vi "Process.vi"(8 "error in":errorcluster, 11 "UI_Main_Test":refnum<class "UI_Main.lvclass">) -> (0 "error out":errorcluster, 3 "UI_Main_Test out":refnum<class "UI_Main.lvclass">)   [LabVIEW 2016, in "UI_Main.lvclass"]
doc: "---------------------------------------------------------------\nJKI State Machine Objects™\nhttp://jki.net/state-machine-objects/\nCopyright (C) 2005-2015, JKI <info@jki.net>\nALL RIGHTS RESERVED"
uses:
  UI_Main.lvclass
  <vilib>/JKI/JKI SMO/SMO/SMO.lvclass
  <vilib>/JKI/JKI SMO/SMO/Typedefs/Parent Call--Enum.ctl
  UI_DAQ_config/UI_DAQ_config.lvclass
  Typedefs/SubUIs.ctl
  UI_Scope/UI_Scope.lvclass
  UI_Generator_Config/UI_Generator_Config.lvclass
  UI_DSP_Config/UI_DSP_Config.lvclass
  lockin/system.lvclass
  C:/Program Files (x86)/National Instruments/LabVIEW 2016/vi.lib/JKI/JKI SMO/SMO/SMO.lvclass
panel:
  in  "config Generator":bool
  in  "Shutdown":bool
  in  "config DSP":bool
  in  "config DAQs":bool
  in  "show Scope":bool
  # "For instructions on how to use the JKI State Machine Objects, examples and video tutorials, visit:\nhttp://jki.net/state-machine-objects/\n\nJKI State Machine Objects™\nhttp://jki.net/state-machine-objects/\nCopyright (C) 2005-2015, JKI <info@jki.net>\nALL RIGHTS RESERVED"
  # "main UI: Always running?"
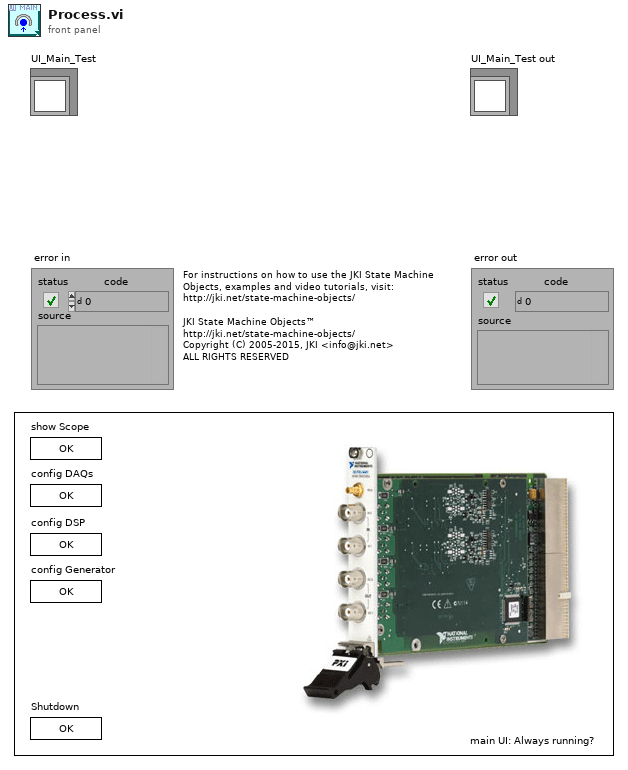
[diagram p1: front panel]
types:
  T1 = typedef "SMO.lvclass/Parent Call--Enum.ctl" = enum16{"Allows parent to run", "Does not request parent to run"}
  T2 = enum32{"invalid app kind", "Development System", "Run Time System", "Student Edition", "Embedded LabVIEW", "Evaluation", "Custom"}
  T3 = enum32{"Invalid", "Standard", "Closed", "Hidden", "Minimized", "Maximized"}
  T4 = enum32{"Bad", "Idle", "Run top level", "Running"}
  T5 = typedef "system.lvclass/Dependencies-cluster.ctl" = cluster{"DAQ_Manager":refnum<class "DAQ_Manager.lvclass">, "DSP":refnum<class "DSP.lvclass">, "Generator":refnum<class "Generator.lvclass">, "Scope":refnum<class "Scope.lvclass">}
  T6 = typedef "UI_Main.lvclass/SubUIs.ctl" = cluster{"UI_DAQ":refnum<class "UI_DAQ_config.lvclass">, "UI_DSP":refnum<class "UI_DSP_Config.lvclass">, "UI_Generator":refnum<class "UI_Generator_Config.lvclass">, "UI_Scope":refnum<class "UI_Scope.lvclass">}
  T7 = cluster{"Core":cluster{"Current VI Reference":refnum<vi>, "Close Panel on Exit?":bool, "error":errorcluster}, "Self Reference":refnum<class "UI_Main.lvclass">, "system":refnum<class "system.lvclass">, "Dependencies":T5, "UIs":T6}
  T8 = cluster{"Current VI Reference":refnum<vi>, "Close Panel on Exit?":bool, "error":errorcluster}
  T9 = typedef "SMO.lvclass/Protected Events.ctl" = cluster{"StopProcesses":refnum<user-event>, "AbortProcesses":refnum<user-event>, "Config Changed":refnum<user-event>, "Dependency":refnum<user-event>}
  T10 = typedef "SMO.lvclass/SMOState --Enum.ctl" = enum16{"unknown", "Created", "Started", "Stopped"}
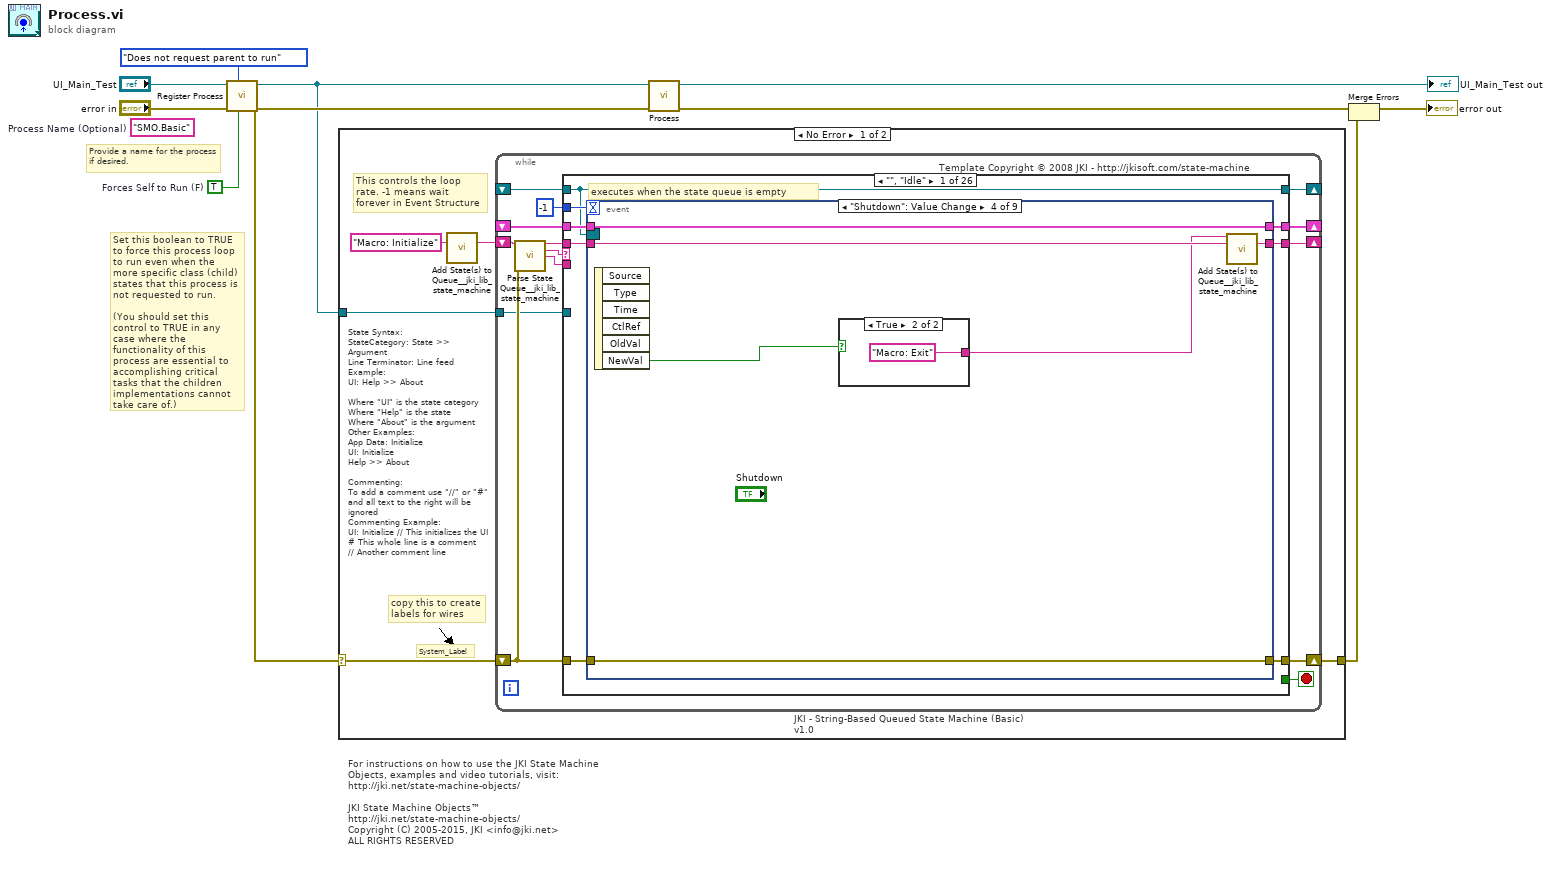
[diagram p0: block diagram]
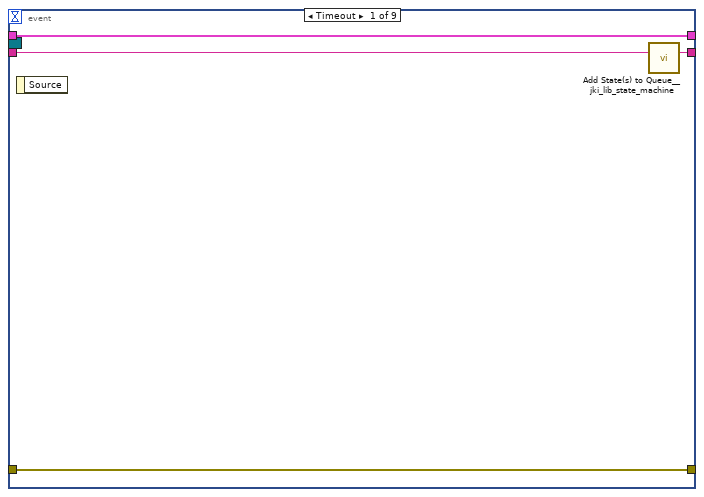
[diagram p2: hidden frame]
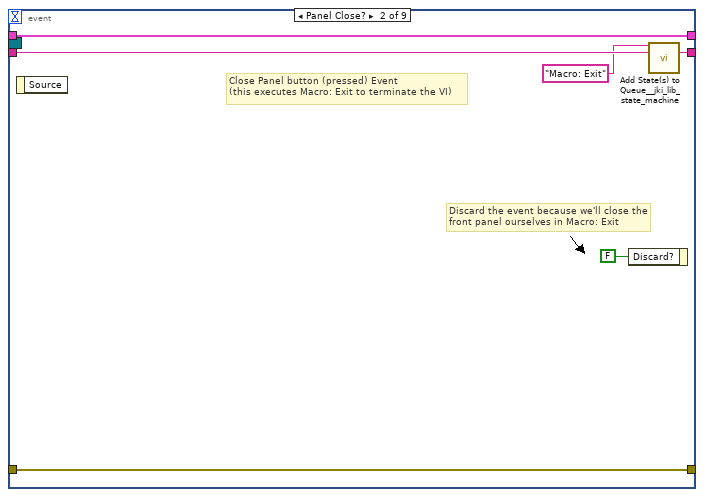
[diagram p3: hidden frame]
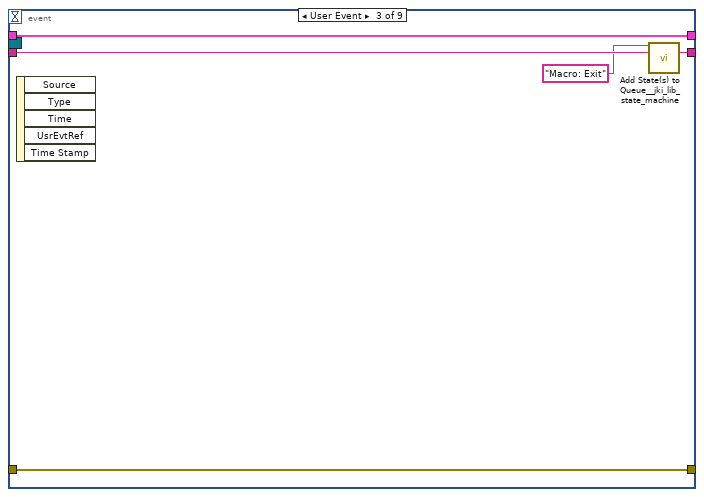
[diagram p4: hidden frame]
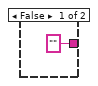
[diagram p5: hidden frame]
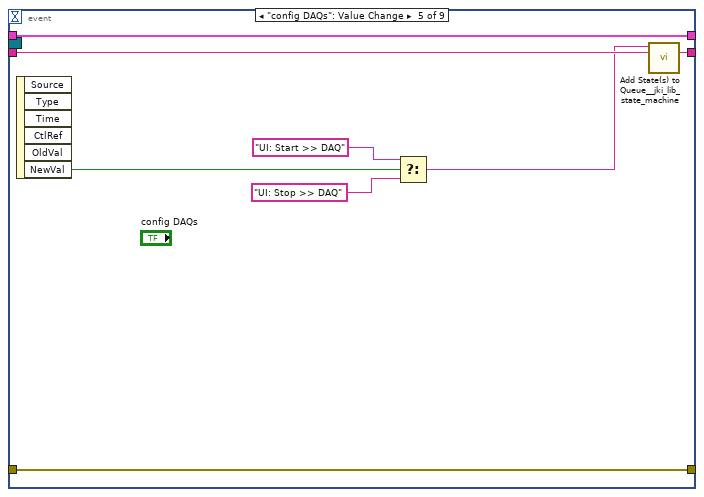
[diagram p6: hidden frame]
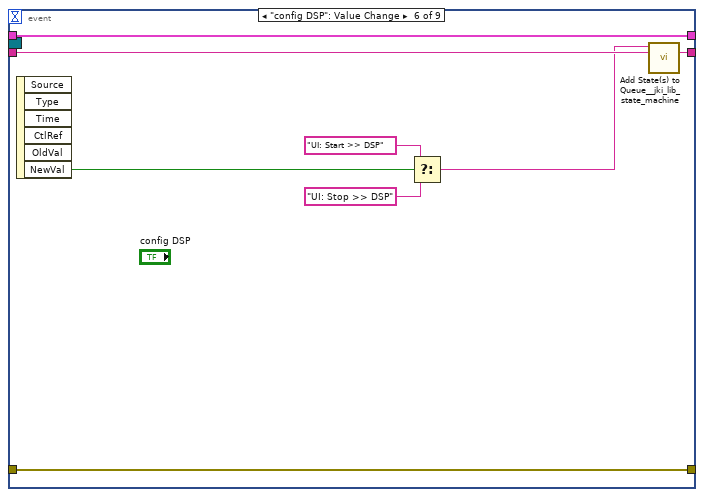
[diagram p7: hidden frame]
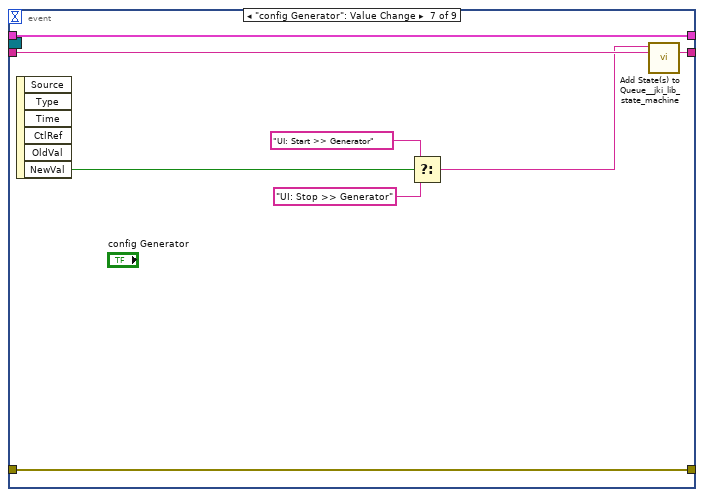
[diagram p8: hidden frame]
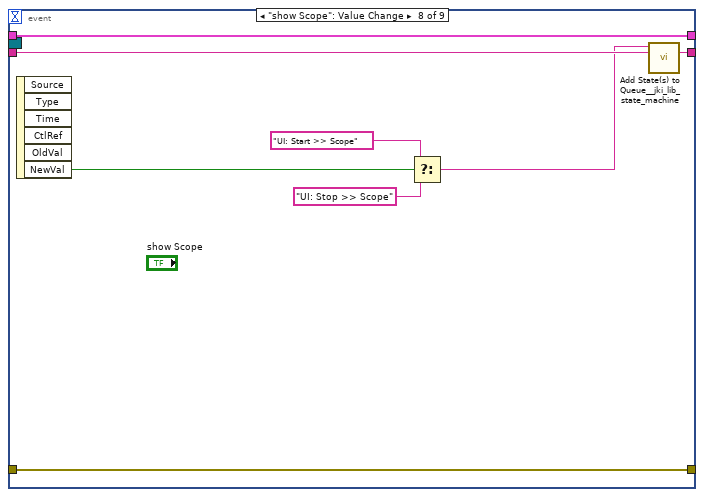
[diagram p9: hidden frame]
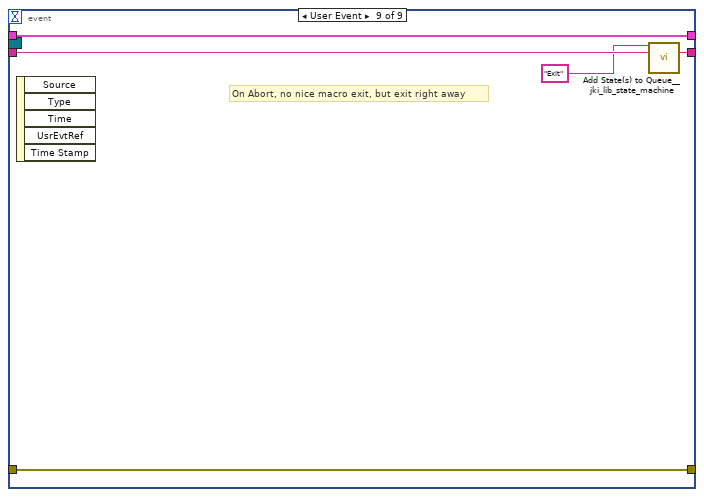
[diagram p10: hidden frame]
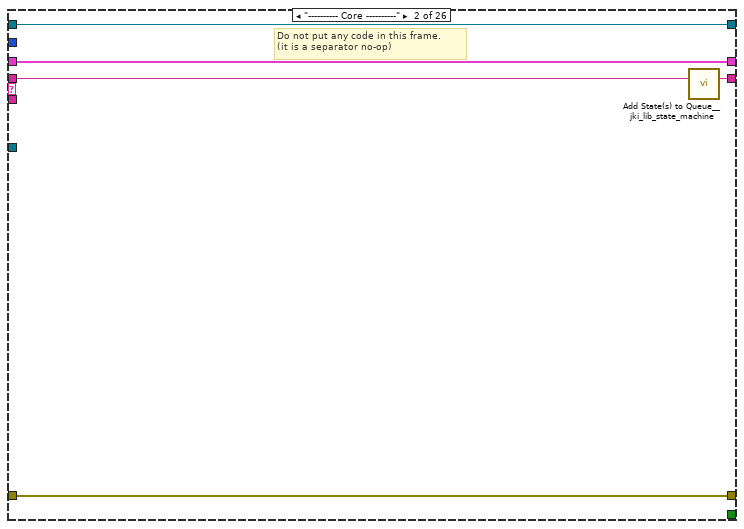
[diagram p11: hidden frame]
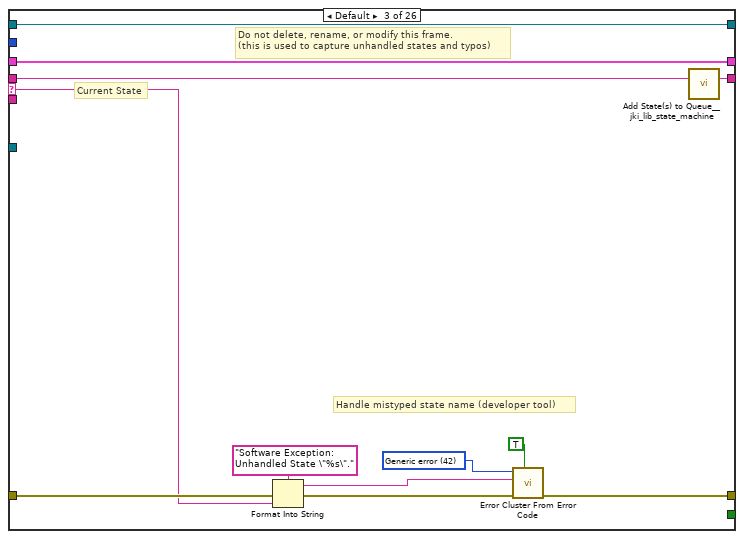
[diagram p12: hidden frame]
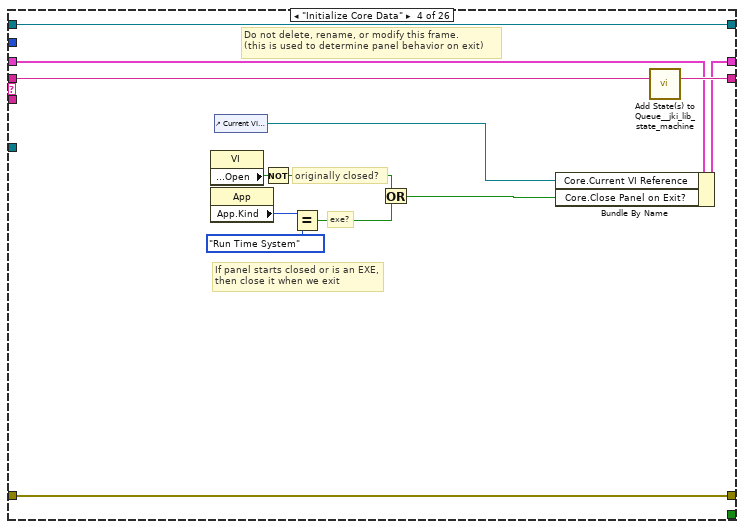
[diagram p13: hidden frame]
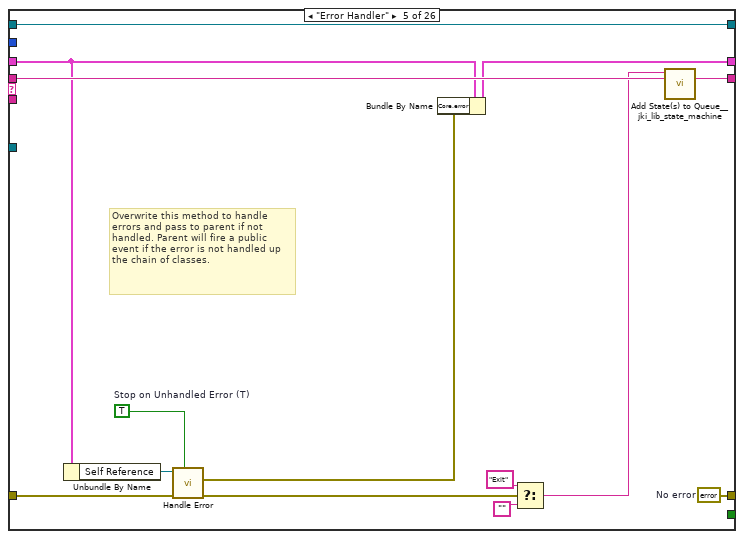
[diagram p14: hidden frame]
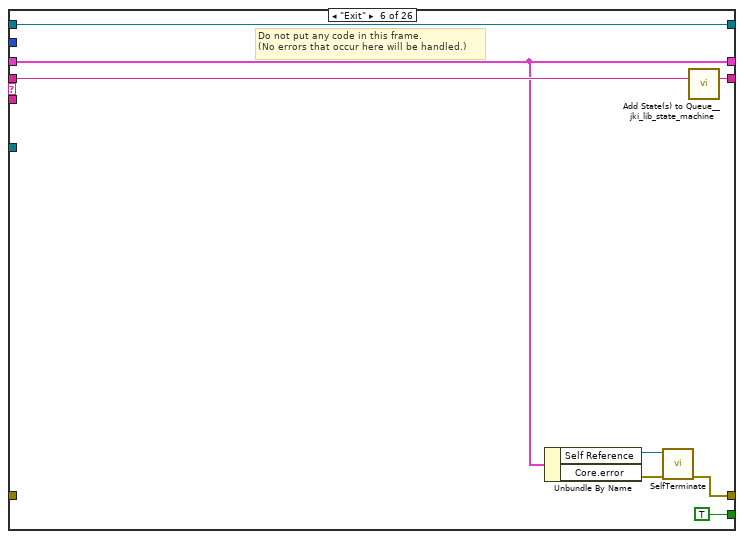
[diagram p15: hidden frame]
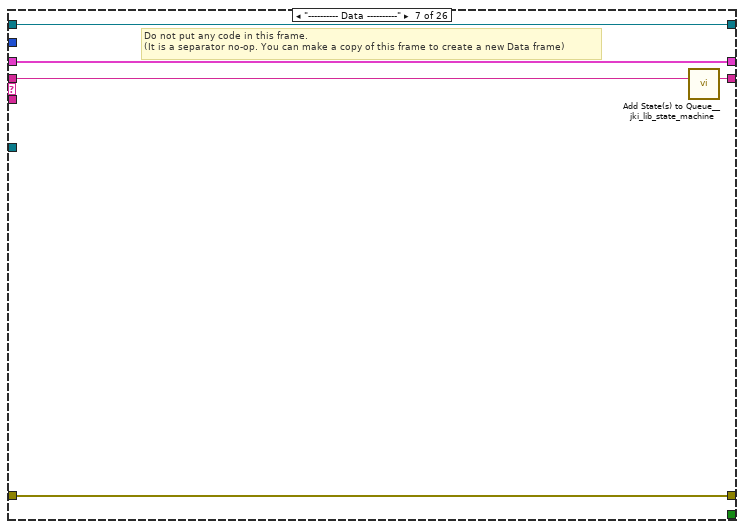
[diagram p16: hidden frame]
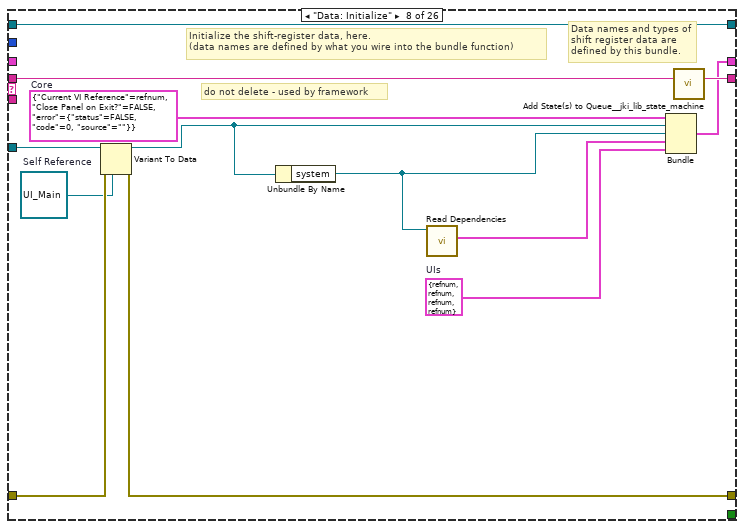
[diagram p17: hidden frame]
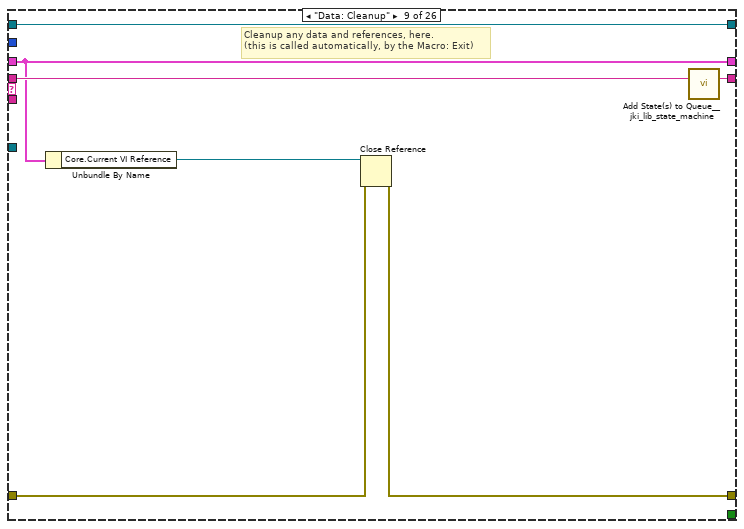
[diagram p18: hidden frame]
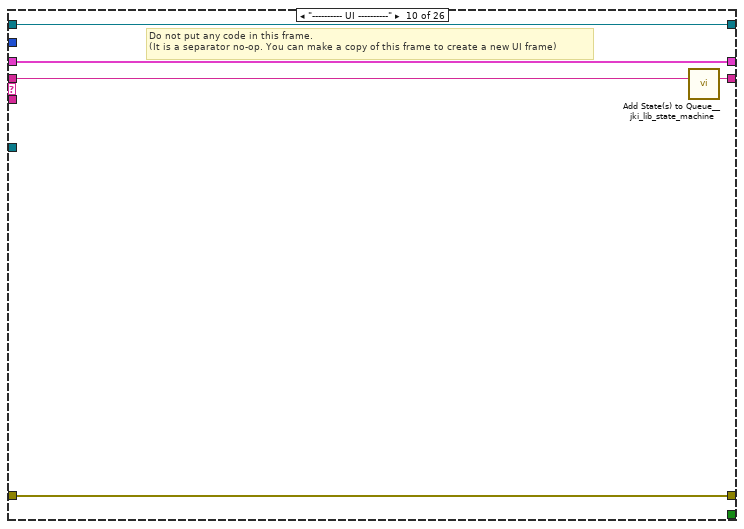
[diagram p19: hidden frame]
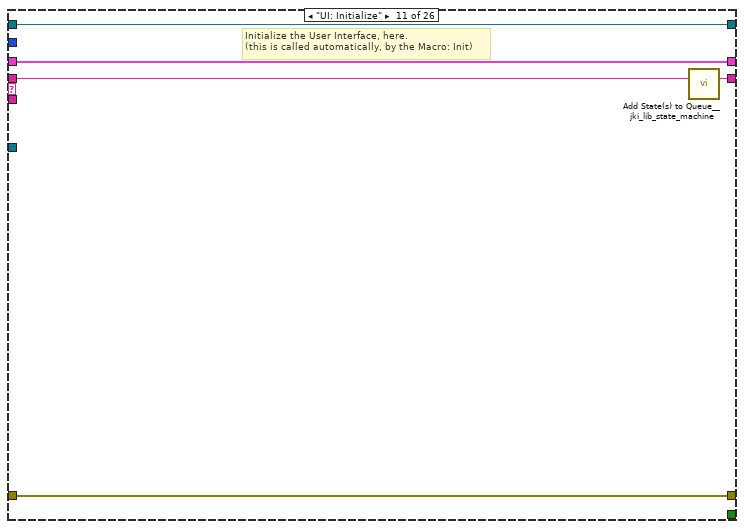
[diagram p20: hidden frame]
diagram:
  w1 = TRUE  # Forces Self to Run (F)
  (unwired) "SMO.Basic"  # Process Name (Optional)
  # "Provide a name for the process\nif desired."
  # "Set this boolean to TRUE to force this process loop to run even when the more specific class (child) states that this process is not requested to run.\n\n(You should set this control to TRUE in any case where the functionality of this process are essential to accomplishing critical tasks that the children implementations cannot take care of.)"
  # "For instructions on how to use the JKI State Machine Objects, examples and video tutorials, visit:\nhttp://jki.net/state-machine-objects/\n\nJKI State Machine Objects™\nhttp://jki.net/state-machine-objects/\nCopyright (C) 2005-2015, JKI <info@jki.net>\nALL RIGHTS RESERVED"
  n1 = call <vilib>:"Register Process.vi"("Forces Self to Run (F)"=w1, "Parent Call"=Parent_Call--Enum."Does not request parent to run", "error in (no error)"="error in", "SMO"="UI_Main_Test") -> ("error out"=w7:errorcluster, "SMO out"=w6:refnum<class "UI_Main.lvclass">)  [unwired: 6 in]
  n2 = case shown="No Error" w7 {
    selector: w7 -> [w12 w383]
    tunnel: w6 -> [w13 _]
    tunnel: [w11 w383] -> w3
    frame No Error {
      # "State Syntax:\nStateCategory: State >> Argument\nLine Terminator: Line feed\nExample:\nUI: Help >> About\n\nWhere \"UI\" is the state category\nWhere \"Help\" is the state\nWhere \"About\" is the argument\nOther Examples:\nApp Data: Initialize\nUI: Initialize\nHelp >> About\n\nCommenting:\nTo add a comment use \"//\" or \"#\" and all text to the right will be ignored\nCommenting Example:\nUI: Initialize // This initializes the UI\n# This whole line is a comment\n// Another comment line"
      # "copy this to create labels for wires"
      # "This controls the loop rate. -1 means wait forever in Event Structure"
      # "System_Label"
      n3 = call <vilib>:"Add State(s) to Queue__jki_lib_state_machine.vi"("State(s) in (\"\")"="Macro: Initialize") -> ("States Out"=w15:string)  [unwired: 14 in]
      n4 = while "JKI - String-Based Queued State Machine (Basic) v1.0" {
        shift-right: [w22] -> _
        shift-left: _ -> [w21]
        shift-right: [w25] -> w11
        shift-left: w12 -> [w19]
        shift-right: [w24] -> _
        shift-left: w15 -> [w26]
        tunnel: w13 -> [w18]
        shift-right: [w17] -> _
        shift-left: _ -> [w16]
        stop <- w23 stop-if-true
        # "Template Copyright © 2008 JKI - http://jkisoft.com/state-machine"
        n5 = call <vilib>:"Parse State Queue__jki_lib_state_machine.vi"("State Queue"=w26, "Error In (no error)"=w19) -> ("Remaining States"=w28:string, "Current State"=w29:string, "Arguments"=w27:string)  [unwired: 11 in]
        n6 = case shown="\"\", \"Idle\"" w29 {
          selector: w29 -> [_ _ w104 _ _ _ _ _ _ _ _ _ _ _ _ _ _ _ _ _ _ _ _ _ _ _]
          tunnel: w28 -> [w37 w102 w108 w127 w141 w149 w154 w167 w174 w179 w184 w191 w207 w239 w253 w267 w272 w283 w288 w298 w304 w309 w328 w340 w356 w368]
          tunnel: w27 -> [_ _ _ _ _ _ _ _ _ _ _ w185 w201 _ _ _ _ _ _ _ _ _ _ w329 w352 _]
          tunnel: w21 -> [w35 w99 w106 w118 w135 w145 w151 _ w169 w176 w182 w189 w203 w236 w249 w258 w269 w280 w285 w296 w302 w307 w325 w336 w351 w365]
          tunnel: [w34 w100 w110 w124 w136 w144 w152 w163 w170 w177 w181 w186 w204 w237 w251 w265 w270 w274 w286 w291 w300 w305 w310 w337 w353 w361] -> w25
          tunnel: w19 -> [w33 w100 w109 w124 w137 _ w152 w164 w171 w177 w181 w187 w205 w237 w251 w265 w270 w275 w286 w292 w300 w305 w311 w333 w348 w364]
          tunnel: [w36 w101 w107 w126 w140 w148 w153 w166 w173 w178 w183 w190 w206 w238 w252 w266 w271 w282 w287 w297 w303 w308 w327 w339 w355 w367] -> w24
          tunnel: [_ _ _ _ _ TRUE _ _ _ _ _ _ _ _ _ _ _ _ _ _ _ _ _ _ _ _] -> w23
          tunnel: [w32 w99 w106 w125 w134 w145 w151 w165 w169 w176 w182 w189 w203 w236 w249 w258 w269 w280 w285 w296 w302 w307 w324 w336 w351 w365] -> w22
          tunnel: -1 ("Timeout") -> [w31 _ _ _ _ _ _ _ _ _ _ _ _ _ _ _ _ _ _ _ _ _ _ _ _ _]
          tunnel: w18 -> [_ _ _ _ _ _ _ w159 _ _ _ _ _ _ _ _ _ _ _ _ _ _ _ _ _ _]
          tunnel: [w30 w98 w103 w115 w139 w146 w150 w161 w168 w175 w180 w188 w200 w235 w250 w259 w268 w281 w284 w295 w301 w306 w326 w338 w354 w366] -> w17
          tunnel: w16 -> [w30 w98 w103 w115 w139 w146 w150 w161 w168 w175 w180 w188 w200 w235 w250 w259 w268 w281 w284 _ w301 w306 w326 w338 w354 w366]
          frame "", "Idle" {
            # "executes when the state queue is empty"
            n7 = event shown="[3] \"Shutdown\": Value Change" {
              selector: w30 -> [_ _ _ _ _ _ _ _ _]
              dyn-events: _ -> [_ _ _ _ _ _ _ _ _]
              timeout: w31 -> [_ _ _ _ _ _ _ _ _]
              tunnel: w37 -> [w41 w47 w52 w58 w68 w76 w84 w92 w97]
              tunnel: [w40 w46 w51 w57 w67 w75 w83 w91 w96] -> w36
              tunnel: w35 -> [w39 w44 w49 w55 w65 w73 w81 w89 w94]
              tunnel: [w38 w45 w50 w56 w66 w74 w82 w90 w95] -> w34
              tunnel: w33 -> [w38 w45 w50 w56 w66 w74 w82 w90 w95]
              tunnel: [w39 w44 w49 w55 w65 w73 w81 w89 w94] -> w32
              event Timeout {
                n8 = event-data() -> ()  [unwired: 1 in, 1 out]
                n9 = call <vilib>:"Add State(s) to Queue__jki_lib_state_machine.vi"("State(s) in (\"\")"=w41) -> ("States Out"=w40:string)  [unwired: 14 in]
              }
              event Panel Close? {
                # "Discard the event because we'll close the front panel ourselves in Macro: Exit"
                # "Close Panel button (pressed) Event\n(this executes Macro: Exit to terminate the VI)"
                n10 = event-data() -> ()  [unwired: 1 in, 1 out]
                n11 = event-data("Discard?"=FALSE) -> ()  [unwired: 1 in, 1 out]
                n12 = call <vilib>:"Add State(s) to Queue__jki_lib_state_machine.vi"("State(s) in Front (\"\")"="Macro: Exit", "State(s) in (\"\")"=w47) -> ("States Out"=w46:string)  [unwired: 13 in]
              }
              event User Event {
                n13 = event-data() -> ()  [unwired: 1 in, 5 out]
                n14 = call <vilib>:"Add State(s) to Queue__jki_lib_state_machine.vi"("State(s) in Front (\"\")"="Macro: Exit", "State(s) in (\"\")"=w52) -> ("States Out"=w51:string)  [unwired: 13 in]
              }
              event "Shutdown": Value Change {
                n15 = event-data() -> ("NewVal"=w53:bool)  [unwired: 1 in, 5 out]
                n16 = case shown="True" w53 {
                  tunnel: ["" "Macro: Exit"] -> w54
                  frame False {
                  }
                  frame True {
                  }
                }
                n17 = call <vilib>:"Add State(s) to Queue__jki_lib_state_machine.vi"("State(s) in Front (\"\")"=w54, "State(s) in (\"\")"=w58) -> ("States Out"=w57:string)  [unwired: 13 in]
              }
              event "config DAQs": Value Change {
                n18 = event-data() -> ("NewVal"=w64:bool)  [unwired: 1 in, 5 out]
                n19 = Select(t="UI: Start >> DAQ", s=w64, f="UI: Stop >> DAQ") -> (s? t:f=w61:string)
                n20 = call <vilib>:"Add State(s) to Queue__jki_lib_state_machine.vi"("State(s) in Front (\"\")"=w61, "State(s) in (\"\")"=w68) -> ("States Out"=w67:string)  [unwired: 13 in]
              }
              event "config DSP": Value Change {
                n21 = event-data() -> ("NewVal"=w72:bool)  [unwired: 1 in, 5 out]
                n22 = Select(t="UI: Start >> DSP", s=w72, f="UI: Stop >> DSP") -> (s? t:f=w71:string)
                n23 = call <vilib>:"Add State(s) to Queue__jki_lib_state_machine.vi"("State(s) in Front (\"\")"=w71, "State(s) in (\"\")"=w76) -> ("States Out"=w75:string)  [unwired: 13 in]
              }
              event "config Generator": Value Change {
                n24 = event-data() -> ("NewVal"=w80:bool)  [unwired: 1 in, 5 out]
                n25 = Select(t="UI: Start >> Generator", s=w80, f="UI: Stop >> Generator") -> (s? t:f=w79:string)
                n26 = call <vilib>:"Add State(s) to Queue__jki_lib_state_machine.vi"("State(s) in Front (\"\")"=w79, "State(s) in (\"\")"=w84) -> ("States Out"=w83:string)  [unwired: 13 in]
              }
              event "show Scope": Value Change {
                n27 = event-data() -> ("NewVal"=w88:bool)  [unwired: 1 in, 5 out]
                n28 = Select(t="UI: Start >> Scope", s=w88, f="UI: Stop >> Scope") -> (s? t:f=w87:string)
                n29 = call <vilib>:"Add State(s) to Queue__jki_lib_state_machine.vi"("State(s) in Front (\"\")"=w87, "State(s) in (\"\")"=w92) -> ("States Out"=w91:string)  [unwired: 13 in]
              }
              event User Event {
                # "On Abort, no nice macro exit, but exit right away"
                n30 = event-data() -> ()  [unwired: 1 in, 5 out]
                n31 = call <vilib>:"Add State(s) to Queue__jki_lib_state_machine.vi"("State(s) in Front (\"\")"="Exit", "State(s) in (\"\")"=w97) -> ("States Out"=w96:string)  [unwired: 13 in]
              }
            }
          }
          frame "---------- Core ----------" {
            # "Do not put any code in this frame.\n(it is a separator no-op)"
            n32 = call <vilib>:"Add State(s) to Queue__jki_lib_state_machine.vi"("State(s) in (\"\")"=w102) -> ("States Out"=w101:string)  [unwired: 14 in]
          }
          frame Default {
            w113 = 42 items=["No error", "Argument error", "Memory is full", "Out of zone", "End of file", "File already open", "Generic file I/O error", "File not found", "File permission error", "Disk is full", "Duplicate path", "Too many files open", "System feature not enabled", "Resource file not found", "Cannot add resource", "Resource not found", "Image not found", "Image memory error", "Pen does not exist", "Config type invalid", "Config token not found", "Config parse error", "Config memory error", "Bad external code format", "Bad external code offset", "External code not present", "Null window", "Destroy window error", "Null menu", "Print aborted", "Bad print record", "Print driver error", "Windows error during printing", "Memory error during printing", "Print dialog error", "Generic print error", "Invalid device refnum", "Device not found", "Device parameter error", "Device unit error", "Cannot open device", "Device call aborted", "Generic error", "Cancelled by user", "Object ID too low", "Object ID too high", "Object not in heap", "Unknown heap", "Unknown object (invalid DefProc)", "Unknown object (DefProc not in table)", "Message out of range", "Invalid (null) method", "Unknown message", "Manager call not supported", "Bad address", "Network operation in progress", "Network operation timed out", "Connection is busy", "Network attribute not supported", "Network error", "Address in use", "System out of memory", "Connection aborted", "Connection refused", "Not connected", "Already connected", "Connection closed", "Initialization error (interapplication manager)", "Bad occurrence", "Wait on unbound occurrence handler", "Occurrence queue overflow", "Datalog type conflict", "Unused", "Unrecognized type (interapplication manager)", "Memory corrupt", "Failed to make temporary DLL", "Old CIN version", "Drag socket not found", "Failed to load drop-object", "Failed to register OLE object", "Failed to release OLE object", "Format specifier type mismatch", "Unknown format specifier", "Too few format specifiers", "Too many format specifiers", "Scan failed", "Newer CIN version", "Error converting to variant", "Runtime menu error", "Password tampered", "Variant attribute not found", "Incompatible variant data type", "Event data is not available", "Event Store is not present", "Occurrence is not found", "Event Queue is not created", "Event info is not available", "Refnum passed is NULL", "Error retrieving Class GUID", "Error retrieving CoClass GUID", "Error retrieving TypeLib GUID.", "Bad built application magic bytes.", "Specific driver is different from the specific driver associated with the Logical Name.", "There is no session opened to the class driver.", "Max Error", "MAX - Error with config objects", "MAX - Error loading configuration", "MAX - Group not supported"]
            # "Current State"
            # "Do not delete, rename, or modify this frame.\n(this is used to capture unhandled states and typos)"
            # "Handle mistyped state name (developer tool)"
            n33 = Format Into String(format string="Software Exception: Unhandled State \"%s\"." ("message"), error in=w109, w104) -> (resulting string=w112:string, error out=w111:errorcluster)  [unwired: 1 in]
            n34 = call <vilib>:"Error Cluster From Error Code.vi"("show call chain? (False)"=TRUE, "error in (no error)"=w111, "error message (\"\")"=w112, "error code (0)"=w113) -> ("error out"=w110:errorcluster)  [unwired: 5 in]
            n35 = call <vilib>:"Add State(s) to Queue__jki_lib_state_machine.vi"("State(s) in (\"\")"=w108) -> ("States Out"=w107:string)  [unwired: 14 in]
          }
          frame "Initialize Core Data" {
            # "Do not delete, rename, or modify this frame.\n(this is used to determine panel behavior on exit)"
            # "originally closed?"
            # "exe?"
            # "If panel starts closed or is an EXE, then close it when we exit"
            n36 = property class="VI"() -> ("Front Panel.Open"=w123:bool)  [unwired: 2 in, 2 out]
            n37 = property class="App"() -> ("App.Kind"=w122:T2)  [unwired: 2 in, 2 out]
            n38 = control-ref of="Current VI Reference"() -> (w116:refnum<vi>)
            n39 = Not(x=w123) -> (.not. x?=w120:bool)
            n40 = Equal?(x=w122, y=T2."Run Time System" ("Application:Kind")) -> (x = y?=w119:bool)
            n41 = Or(x=w120, y=w119) -> (x .or. y?=w117:bool)
            n42 = Bundle By Name(cluster=w118, "Core.Current VI Reference"=w116, "Core.Close Panel on Exit?"=w117) -> (w125:T7)
            n43 = call <vilib>:"Add State(s) to Queue__jki_lib_state_machine.vi"("State(s) in (\"\")"=w127) -> ("States Out"=w126:string)  [unwired: 14 in]
          }
          frame "Error Handler" {
            w128 = TRUE  # Stop on Unhandled Error (T)
            w136 = errorcluster {"status"=FALSE, "code"=0, "source"=""}  # No error
            # "Overwrite this method to handle errors and pass to parent if not handled. Parent will fire a public event if the error is not handled up the chain of classes."
            n44 = Unbundle By Name(w135) -> ("Self Reference"=w138:refnum<class "UI_Main.lvclass">)
            n45 = call-dynamic "Handle Error.vi"("Stop on Unhandled Error (T)"=w128, "error in"=w137, "SMO"=w138) -> ("handling error"=w129:errorcluster, "Unhandled error"=w132:errorcluster)  [unwired: 6 in, 1 out]
            n46 = Bundle By Name(cluster=w135, "Core.error"=w132) -> (w134:T7)
            n47 = Select(t="Exit", s=w129, f="") -> (s? t:f=w133:string)
            n48 = call <vilib>:"Add State(s) to Queue__jki_lib_state_machine.vi"("State(s) in Front (\"\")"=w133, "State(s) in (\"\")"=w141) -> ("States Out"=w140:string)  [unwired: 13 in]
          }
          frame "Exit" {
            # "Do not put any code in this frame.\n(No errors that occur here will be handled.)"
            n49 = Unbundle By Name(w145) -> ("Self Reference"=w143:refnum<class "UI_Main.lvclass">, "Core.error"=w142:errorcluster)
            n50 = call <vilib>:"SelfTerminate.vi"("error in (no error)"=w142, "SMO in"=w143) -> ("error out"=w144:errorcluster)  [unwired: 8 in, 1 out]
            n51 = call <vilib>:"Add State(s) to Queue__jki_lib_state_machine.vi"("State(s) in (\"\")"=w149) -> ("States Out"=w148:string)  [unwired: 14 in]
          }
          frame "---------- Data ----------" {
            # "Do not put any code in this frame.\n(It is a separator no-op. You can make a copy of this frame to create a new Data frame)"
            n52 = call <vilib>:"Add State(s) to Queue__jki_lib_state_machine.vi"("State(s) in (\"\")"=w154) -> ("States Out"=w153:string)  [unwired: 14 in]
          }
          frame "Data: Initialize" {
            w156 = T6 {"UI_DAQ"=refnum, "UI_DSP"=refnum, "UI_Generator"=refnum, "UI_Scope"=refnum}  # UIs
            w160 = T8 {"Current VI Reference"=refnum, "Close Panel on Exit?"=FALSE, "error"={"status"=FALSE, "code"=0, "source"=""}}  # Core
            w162 = refnum<class "UI_Main.lvclass"> refnum  # Self Reference
            # "do not delete - used by framework"
            # "Data names and types of shift register data are defined by this bundle."
            # "Initialize the shift-register data, here.\n(data names are defined by what you wire into the bundle function)"
            n53 = Variant To Data(error in=w164, type=w162, Variant=w159) -> (data=w155:refnum<class "UI_Main.lvclass">, error out=w163:errorcluster)
            n54 = Unbundle By Name(w155) -> ("system"=w158:refnum<class "system.lvclass">)
            n55 = call "Read Dependencies.vi"("system in"=w158) -> ("Dependencies"=w157:T5)  [unwired: 8 in, 2 out]
            n56 = Bundle("Core"=w160, "Self Reference"=w155, "system"=w158, "Dependencies"=w157, "UIs"=w156) -> (w165:T7)  [unwired: 1 in]
            n57 = call <vilib>:"Add State(s) to Queue__jki_lib_state_machine.vi"("State(s) in (\"\")"=w167) -> ("States Out"=w166:string)  [unwired: 14 in]
          }
          frame "Data: Cleanup" {
            # "Cleanup any data and references, here.\n(this is called automatically, by the Macro: Exit)"
            n58 = Unbundle By Name(w169) -> ("Core.Current VI Reference"=w172:refnum<vi>)
            n59 = Close Reference(reference=w172, error in (no error)=w171) -> (error out=w170:errorcluster)
            n60 = call <vilib>:"Add State(s) to Queue__jki_lib_state_machine.vi"("State(s) in (\"\")"=w174) -> ("States Out"=w173:string)  [unwired: 14 in]
          }
          frame "---------- UI ----------" {
            # "Do not put any code in this frame.\n(It is a separator no-op. You can make a copy of this frame to create a new UI frame)"
            n61 = call <vilib>:"Add State(s) to Queue__jki_lib_state_machine.vi"("State(s) in (\"\")"=w179) -> ("States Out"=w178:string)  [unwired: 14 in]
          }
          frame "UI: Initialize" {
            # "Initialize the User Interface, here.\n(this is called automatically, by the Macro: Init)"
            n62 = call <vilib>:"Add State(s) to Queue__jki_lib_state_machine.vi"("State(s) in (\"\")"=w184) -> ("States Out"=w183:string)  [unwired: 14 in]
          }
          frame "UI: Cursor Set" {
            # "Argument"
            # "Initialize the User Interface, here.\n(this is called automatically, by the Macro: Init)"
            n63 = disable-structure shown="Default" {
              disable-tunnel: w187 -> [w192 w195]
              disable-tunnel: [w192 w194] -> w186
              disable-tunnel: w185 -> [_ w193]
              frame condition #0 {
              }
              frame condition #1 (active) {
                n64 = case shown="\"Idle\", Default" w193 {
                  tunnel: w195 -> [w197 w199]
                  tunnel: [w196 w198] -> w194
                  frame "Idle", Default {
                    n65 = call <vilib>:"Unset Busy.vi"("error in (no error)"=w197) -> ("error out"=w196:errorcluster)  [unwired: 10 in]
                  }
                  frame "Busy" {
                    n66 = call <vilib>:"Set Busy.vi"("error in (no error)"=w199) -> ("error out"=w198:errorcluster)  [unwired: 9 in, 1 out]
                  }
                }
              }
            }
            n67 = call <vilib>:"Add State(s) to Queue__jki_lib_state_machine.vi"("State(s) in (\"\")"=w191) -> ("States Out"=w190:string)  [unwired: 14 in]
          }
          frame "UI: Front Panel State" {
            # "Argument"
            # "Set Front Panel Open or Closed\n(Usage: \"UI: Front Panel State >> Open|Close\")"
            n68 = Unbundle By Name(w203) -> ("Core.Current VI Reference"=w202:refnum<vi>)
            n69 = disable-structure shown="Default" {
              disable-tunnel: w205 -> [w211 w234]
              disable-tunnel: [w210 w234] -> w204
              disable-tunnel: w202 -> [w209 _]
              disable-tunnel: w201 -> [w208 _]
              frame condition #0 (active) {
                n70 = case shown="\"Close\"" w208 {
                  tunnel: w211 -> [w215 w228]
                  tunnel: [w217 w229] -> w210
                  tunnel: w209 -> [w216 w226]
                  frame "Open", Default {
                    n71 = property class="VI"(reference=w216, error in=w215) -> (reference out=w213:refnum<vi>, error out=w214:errorcluster, "FP.State"=w212:T3)
                    n72 = case shown="\"Closed\"" w212 {
                      tunnel: [w220 w223] -> w217
                      tunnel: w214 -> [w219 w223]
                      tunnel: w213 -> [w218 _]
                      frame "Closed" {
                        n73 = invoke class="VI" method="FP.Open"(reference=w218, error in=w219, "Activate"=TRUE, "State"=T3."Standard") -> (error out=w220:errorcluster)  [unwired: 1 in, 4 out]
                      }
                      frame Default {
                      }
                    }
                  }
                  frame "Close" {
                    n74 = property class="VI"(reference=w226, error in=w228) -> (reference out=w225:refnum<vi>, error out=w227:errorcluster, "FP.State"=w224:T3)
                    n75 = case shown="Default" w224 {
                      tunnel: [w230 w233] -> w229
                      tunnel: w227 -> [w230 w232]
                      tunnel: w225 -> [_ w231]
                      frame "Invalid", "Closed" {
                      }
                      frame Default {
                        n76 = invoke class="VI" method="FP.Close"(reference=w231, error in=w232) -> (error out=w233:errorcluster)  [unwired: 1 in, 2 out]
                      }
                    }
                  }
                }
              }
              frame condition #1 {
              }
            }
            n77 = call <vilib>:"Add State(s) to Queue__jki_lib_state_machine.vi"("State(s) in (\"\")"=w207) -> ("States Out"=w206:string)  [unwired: 14 in]
          }
          frame "---------- Macro ----------" {
            # "Do not put any code in this frame.\n(It is a separator no-op. You can make a copy of this frame to create a new Macro frame)"
            n78 = call <vilib>:"Add State(s) to Queue__jki_lib_state_machine.vi"("State(s) in (\"\")"=w239) -> ("States Out"=w238:string)  [unwired: 14 in]
          }
          frame "Macro: Initialize" {
            w244 = "UI: Initialize\nUI: Front Panel State >> Open"  # UI: Initialize UI: Front Panel State >> Open
            w240 = "Process: Sync"
            # "Initialization Macro\n(This is called once, when the VI starts)"
            n79 = control-ref of="This VI"() -> (w242:refnum<vi>)
            n80 = property class="VI"(reference=w242) -> ("Exec.State"=w241:T4)  [unwired: 1 in, 2 out]
            n81 = Equal?(x=w241, y=T4."Run top level") -> (x = y?=w247:bool)
            n82 = Select(t=w240, s=w247, f="") -> ()  [unwired: 1 out]
            n83 = call <vilib>:"Add State(s) to Queue__jki_lib_state_machine.vi"("State(s) in Front (\"\")"="Data: Initialize\nInitialize Core Data\nEvents: Register\nUI: Create", "State(s) in (\"\")"=w240, "State(s) at Back (\"\")"=w244) -> ("States Out"=w243:string)  [unwired: 12 in]
            n84 = call <vilib>:"Add State(s) to Queue__jki_lib_state_machine.vi"("State(s) in Front (\"\")"=w243, "State(s) in (\"\")"=w253) -> ("States Out"=w252:string)  [unwired: 13 in]
          }
          frame "Macro: Exit" {
            # "Exit Macro\n(This is called once, when the VI exits)"
            n85 = Unbundle By Name(w258) -> ("Core.Close Panel on Exit?"=w264:bool)
            n86 = Select(t="UI: Front Panel State >> Close", s=w264, f="") -> (s? t:f=w261:string)
            n87 = call <vilib>:"Add State(s) to Queue__jki_lib_state_machine.vi"("State(s) in Front (\"\")"="UI: Destroy\nData: Cleanup\nEvents: Unregister", "State(s) in (\"\")"="Process: Sync", "State(s) at Back (\"\")"="Exit") -> ("States Out"=w255:string)  [unwired: 12 in]
            n88 = call <vilib>:"Add State(s) to Queue__jki_lib_state_machine.vi"("State(s) in (\"\")"=w261, "State(s) at Back (\"\")"=w255) -> ("States Out"=w260:string)  [unwired: 13 in]
            n89 = call <vilib>:"Add State(s) to Queue__jki_lib_state_machine.vi"("State(s) in Front (\"\")"=w260, "State(s) in (\"\")"=w267) -> ("States Out"=w266:string)  [unwired: 13 in]
          }
          frame "---------- Process ----------" {
            # "Template Separator\n(You can make a copy of, or modify, this frame)"
            n90 = call <vilib>:"Add State(s) to Queue__jki_lib_state_machine.vi"("State(s) in (\"\")"=w272) -> ("States Out"=w271:string)  [unwired: 14 in]
          }
          frame "Process: Sync" {
            n91 = Unbundle By Name(w280) -> ("Self Reference"=w276:refnum<class "UI_Main.lvclass">)
            n92 = call <vilib>:"WaitOnProcessSync.vi"("error in (no error)"=w275, "SMO"=w276) -> ("error out"=w274:errorcluster, "Don't run?"=w279:bool)  [unwired: 7 in, 1 out]
            n93 = Select(t="Data: Cleanup\nEvents: Unregister\nExit", s=w279, f="") -> (s? t:f=w273:string)
            n94 = call <vilib>:"Add State(s) to Queue__jki_lib_state_machine.vi"("State(s) in Front (\"\")"=w273, "State(s) in (\"\")"=w283) -> ("States Out"=w282:string)  [unwired: 13 in]
          }
          frame "---------- Events ----------" {
            # "Template Separator\n(You can make a copy of, or modify, this frame)"
            n95 = call <vilib>:"Add State(s) to Queue__jki_lib_state_machine.vi"("State(s) in (\"\")"=w288) -> ("States Out"=w287:string)  [unwired: 14 in]
          }
          frame "Events: Register" {
            # "Expand to add\nmore events"
            n96 = Unbundle By Name(w296) -> ("Self Reference"=w293:refnum<class "UI_Main.lvclass">)
            n97 = call <vilib>:"GetProtectedEvents.vi"("SMO"=w293) -> ("error out"=w289:errorcluster, "SMO Protected Events"=w294:T9)  [unwired: 8 in, 1 out]
            n98 = register-events(w294) -> (reference out=w295:refnum<event-registration>, error out=w290:errorcluster)  [unwired: 2 in]
            n99 = Merge Errors(w292, w290, w289) -> (w291:errorcluster)
            n100 = call <vilib>:"Add State(s) to Queue__jki_lib_state_machine.vi"("State(s) in (\"\")"=w298) -> ("States Out"=w297:string)  [unwired: 14 in]
          }
          frame "Events: Unregister" {
            n101 = Unregister For Events(event registration refnum=w301, error in=w300) -> (error out=w299:errorcluster)
            n102 = call <vilib>:"Clear Errors.vi"("error in (no error)"=w299) -> ()  [unwired: 5 in, 2 out]
            n103 = call <vilib>:"Add State(s) to Queue__jki_lib_state_machine.vi"("State(s) in (\"\")"=w304) -> ("States Out"=w303:string)  [unwired: 14 in]
          }
          frame "---------- Action ----------" {
            n104 = call <vilib>:"Add State(s) to Queue__jki_lib_state_machine.vi"("State(s) in (\"\")"=w309) -> ("States Out"=w308:string)  [unwired: 14 in]
          }
          frame "UI: Create" {
            n105 = Unbundle By Name(w325) -> ("UIs.UI_DAQ"=w322:refnum<class "UI_DAQ_config.lvclass">, "UIs.UI_DSP"=w321:refnum<class "UI_DSP_Config.lvclass">, "UIs.UI_Generator"=w320:refnum<class "UI_Generator_Config.lvclass">, "UIs.UI_Scope"=w319:refnum<class "UI_Scope.lvclass">)
            n106 = call "Create UI_DAQ_config.vi"("error in (no error)"=w311, "DAQ_config_UI in"=w322) -> ("error out"=w315:errorcluster, "DAQ_config_UI out"=w323:refnum<class "UI_DAQ_config.lvclass">)  [unwired: 8 in]
            n107 = call "Create UI_DSP_config.vi"("error in (no error)"=w311, "UI_DSP_Config.lvclass"=w321) -> ("error out"=w314:errorcluster, "output cluster"=w318:refnum<class "UI_DSP_Config.lvclass">)  [unwired: 8 in]
            n108 = call "Create UI_Generator_config.vi"("error in (no error)"=w311, "UI_Generator_Config"=w320) -> ("error out"=w313:errorcluster, "UI_Generator_Config"=w317:refnum<class "UI_Generator_Config.lvclass">)  [unwired: 8 in]
            n109 = call "Create UI_Scope.vi"("error in (no error)"=w311, "UI_Scope.lvclass"=w319) -> ("error out"=w312:errorcluster, "UI_Scope.lvclass"=w316:refnum<class "UI_Scope.lvclass">)  [unwired: 8 in]
            n110 = Merge Errors(w315, w314, w313, w312) -> (w310:errorcluster)
            n111 = Bundle By Name(cluster=w325, "UIs.UI_DAQ"=w323, "UIs.UI_DSP"=w318, "UIs.UI_Generator"=w317, "UIs.UI_Scope"=w316) -> (w324:T7)
            n112 = call <vilib>:"Add State(s) to Queue__jki_lib_state_machine.vi"("State(s) in (\"\")"=w328) -> ("States Out"=w327:string)  [unwired: 14 in]
          }
          frame "UI: Start" {
            n113 = Unbundle By Name(w336) -> ("UIs"=w331:T6)
            n114 = call "ParseSubUIs.vi"("Arguments"=w329, "UIs"=w331) -> ("UI_#"=w330:refnum<class "SMO.lvclass">)  [unwired: 9 in]
            n115 = call <vilib>:"GetState.vi"("error in (no error)"=w333, "SMO"=w330) -> ("error out"=w332:errorcluster, "SMO State"=w334:T10, "SMO out"=w335:refnum<class "SMO.lvclass">)  [unwired: 7 in]
            n116 = case shown="\"Created\", \"Stopped\"" w334 {
              tunnel: [w341 w344] -> w337
              tunnel: w335 -> [_ w343]
              tunnel: w332 -> [w341 w342]
              frame Default {
              }
              frame "Created", "Stopped" {
                n117 = call <vilib>:"Start.vi"("error in (no error)"=w342, "SMO"=w343) -> ("error out"=w344:errorcluster)  [unwired: 8 in, 1 out]
              }
            }
            n118 = call <vilib>:"Add State(s) to Queue__jki_lib_state_machine.vi"("State(s) in (\"\")"=w340) -> ("States Out"=w339:string)  [unwired: 14 in]
          }
          frame "UI: Stop" {
            n119 = Unbundle By Name(w351) -> ("UIs"=w350:T6)
            n120 = call "ParseSubUIs.vi"("Arguments"=w352, "UIs"=w350) -> ("UI_#"=w349:refnum<class "SMO.lvclass">)  [unwired: 9 in]
            n121 = call <vilib>:"GetState.vi"("error in (no error)"=w348, "SMO"=w349) -> ("error out"=w347:errorcluster, "SMO State"=w345:T10, "SMO out"=w346:refnum<class "SMO.lvclass">)  [unwired: 7 in]
            n122 = case shown="\"Started\"" w345 {
              tunnel: [w357 w360] -> w353
              tunnel: w347 -> [w357 w359]
              tunnel: w346 -> [_ w358]
              frame Default {
              }
              frame "Started" {
                n123 = call <vilib>:"Stop.vi"("error in (no error)"=w359, "SMO"=w358) -> ("error out"=w360:errorcluster)  [unwired: 8 in, 1 out]
              }
            }
            n124 = call <vilib>:"Add State(s) to Queue__jki_lib_state_machine.vi"("State(s) in (\"\")"=w356) -> ("States Out"=w355:string)  [unwired: 14 in]
          }
          frame "UI: Destroy" {
            n125 = Unbundle By Name(w365) -> ("UIs"=w362:T6)
            n126 = Cluster To Array(cluster=w362) -> (array=w363:refnum<class "SMO.lvclass">[])
            n127 = for {
              tunnel: w363 -> [w372] mode=indexing
              shift-right: [w374] -> w361
              shift-left: w364 -> [w373]
              n128 = call <vilib>:"GetState.vi"("error in (no error)"=w373, "SMO"=w372) -> ("error out"=w369:errorcluster, "SMO State"=w371:T10, "SMO out"=w370:refnum<class "SMO.lvclass">)  [unwired: 7 in]
              n129 = case shown="\"Started\"" w371 {
                tunnel: [w376 w382] -> w374
                tunnel: w370 -> [w375 w379]
                tunnel: w369 -> [w377 w378]
                frame Default {
                  n130 = call <vilib>:"Destroy.vi"("error in (no error)"=w377, "SMO"=w375) -> ("error out"=w376:errorcluster)  [unwired: 9 in]
                }
                frame "Started" {
                  n131 = call <vilib>:"Stop.vi"("error in (no error)"=w378, "SMO"=w379) -> ("error out"=w381:errorcluster, "SMO out"=w380:refnum<class "SMO.lvclass">)  [unwired: 8 in]
                  n132 = call <vilib>:"Destroy.vi"("error in (no error)"=w381, "SMO"=w380) -> ("error out"=w382:errorcluster)  [unwired: 9 in]
                }
              }
            }
            n133 = call <vilib>:"Add State(s) to Queue__jki_lib_state_machine.vi"("State(s) in (\"\")"=w368) -> ("States Out"=w367:string)  [unwired: 14 in]
          }
        }
      }
    }
    frame Error {
    }
  }
  n134 = call-parent "Process.vi"("error in"=w7, "SMO"=w6) -> ("error out"=w4:errorcluster, "SMO out"=→"UI_Main_Test out":refnum<class "UI_Main.lvclass">)  [unwired: 8 in]
  n135 = Merge Errors(w4, w3) -> (→"error out":errorcluster)
